vi "Read Results Queue Table.vi"(8 "error in (no error)":errorcluster, 11 "TestStand Controller in":refnum<class "Controller API.lvclass">) -> (0 "error out":errorcluster, 2 "Results Queue Table":variant, 3 "TestStand Controller out":refnum<class "Controller API.lvclass">)   [LabVIEW 2013, in "Controller API.lvlib" / "Controller API.lvclass"]
uses:
  Controller API.lvclass
  Controller API.lvclass/Controller API.ctl
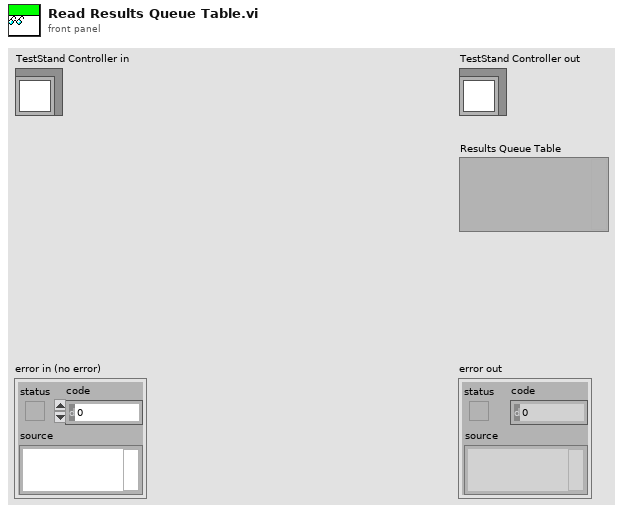
[diagram p1: front panel]
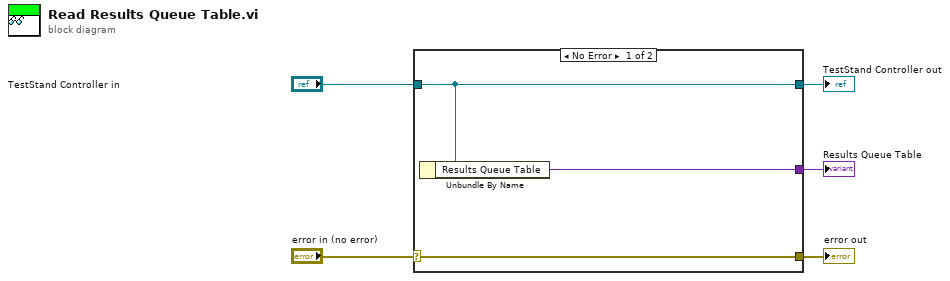
[diagram p0: block diagram]
diagram:
  n1 = case shown="No Error" "error in (no error)" {
    selector: "error in (no error)" -> [w8 w9]
    tunnel: [w8 w9] -> w4
    tunnel: [w7 w10] -> w2
    tunnel: "TestStand Controller in" -> [w7 w10]
    tunnel: [w6 _] -> w1
    frame No Error {
      n2 = Unbundle By Name(w7) -> ("Results Queue Table"=w6:variant)
    }
    frame Error {
    }
  }
  "error out" <- w4
  "TestStand Controller out" <- w2
  "Results Queue Table" <- w1
